vi "RefMem DMA Main Page.vi"(8 "error in (no error)":errorcluster, 11 "Node Ptr":T1 format="%.0x") -> (0 "error out":errorcluster)   [LabVIEW 2015, in "RefMem DMA Custom Device.lvlib"]
uses:
  RefMem DMA Custom Device.lvlib
  <vilib>/NI Veristand/Custom Device API/Custom Device Item Ref.ctl
  <vilib>/NI Veristand/Custom Device API/Custom Device Execution Mode.ctl
  <vilib>/NI Veristand/Custom Device API/Path Specification.ctl
  <vilib>/NI Veristand/Custom Device API/Path Type.ctl
  <vilib>/NI Veristand/Custom Device API/Custom Device Channel.ctl
  <vilib>/NI Veristand/Custom Device API/Custom Device Channel Type.ctl
  Controls/Data Channel Type.ctl
  Reflective Memory File/Reflective Memory File.lvclass
  Controls/Global.vi
  <vilib>/NI Veristand/Custom Device API/Get Item Property (String).vi
  <vilib>/NI Veristand/Custom Device API/Set Item Property (String).vi
  <vilib>/NI Veristand/Custom Device API/Get Item Property (I32).vi
  <vilib>/NI Veristand/Custom Device API/Set Item Property (I32).vi
  <vilib>/NI Veristand/Custom Device API/Set Item Property (U16).vi
  <vilib>/NI Veristand/Custom Device API/Set Item Property (U32).vi
  <vilib>/NI Veristand/Custom Device API/Custom Device API.lvlib
  <vilib>/NI/NI VeriStand Custom Device Import and Export Tool/ImportExport.lvlib
panel:
  out "Path":string
  in  "CPU Assignment":i32
  in  "Import":bool
  in  "Decimation":i32=1 min=1
  in  "VISA Name":string
  in  "Add Data Channel":bool
  in  "Add Data Folder":bool
  in  "Header":cluster{"Section Name":string}={"Section Name"="Reflective Memory Settings"}
  in  "Description":string
  in  "Name":string
  # "(-2 is Automatic)"
  # "Valid values -2, 0, 1.."
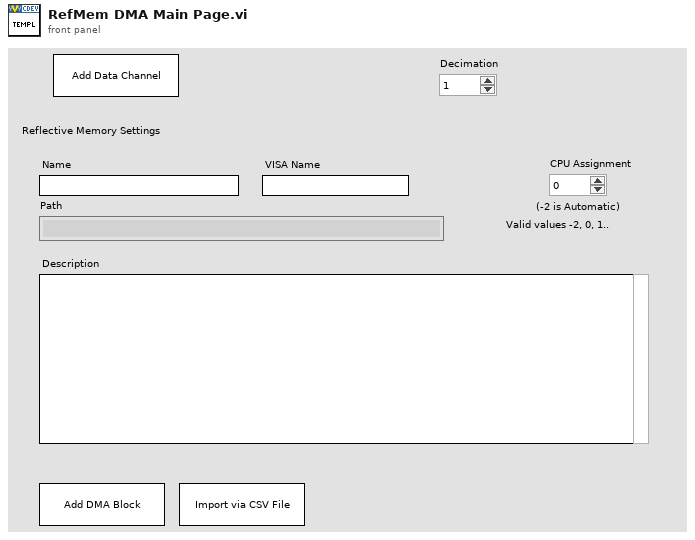
[diagram p1: front panel]
types:
  T1 = typedef "Custom Device API.lvlib/Custom Device Item Ref.ctl" = u64
  T2 = enum8{"Enabled", "Disabled", "Disabled and Grayed Out"}
  T3 = typedef "Custom Device API.lvlib/Custom Device Item Info.ctl" = cluster{"Name":string, "Is Channel":bool, "GUID":string, "Is Waveform":bool}
  T4 = typedef "Custom Device API.lvlib/Path Specification.ctl" = cluster{"Path":path, "Type":T5}
  T5 = typedef "Custom Device API.lvlib/Path Type.ctl" = enum16{"Absolute", "To Base", "To Common Data Dir", "To Application Data Dir"}
  T6 = typedef "Custom Device API.lvlib/Custom Device Execution Mode.ctl" = enum16{"Asynchronous", "Inline HW Interface", "Inline Model Interface", "Inline Timing and Sync", "Asynchronous Timing and Sync"}
  T7 = typedef "RefMem DMA Custom Device.lvlib/Data Channel Type.ctl" = enum16{"Read", "Write"}
  T8 = typedef "Custom Device API.lvlib/Custom Device Channel.ctl" = cluster{"Type":T9, "Units":string, "Default Value":dbl, "Faultable":bool, "Scalable":bool}
  T9 = typedef "Custom Device API.lvlib/Custom Device Channel Type.ctl" = enum16{"Input", "Output"}
  T10 = typedef "Custom Device API.lvlib/Custom Device Commands.ctl" = enum16{"Default", "Item renamed", "Shutdown", "Dynamic button pressed"}
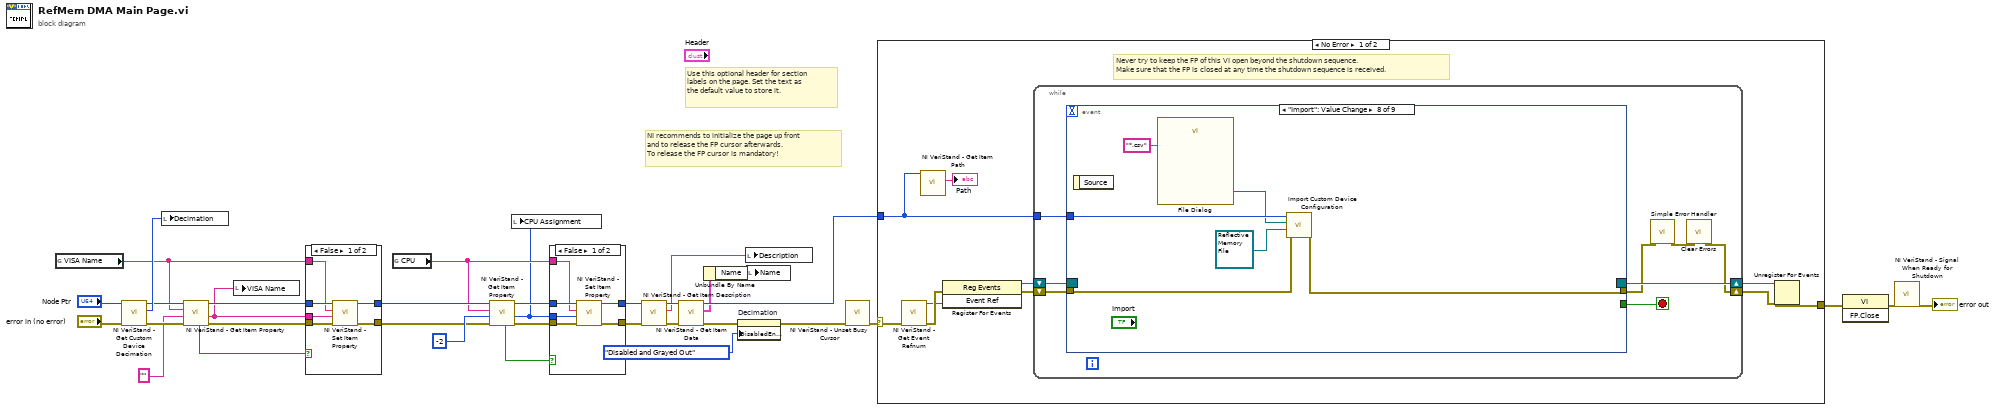
[diagram p0: block diagram]
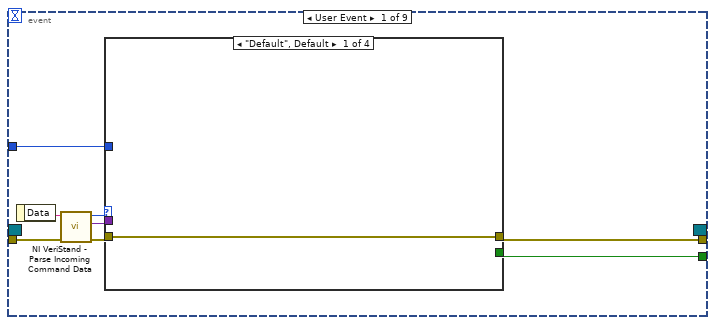
[diagram p4: hidden frame]
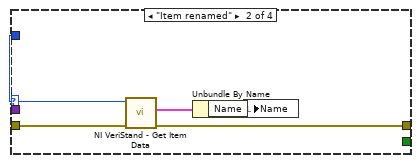
[diagram p5: hidden frame]
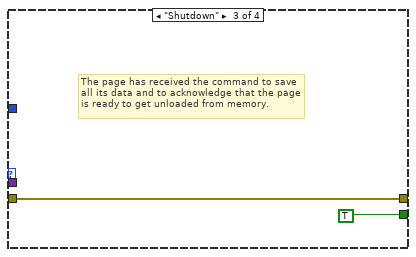
[diagram p6: hidden frame]
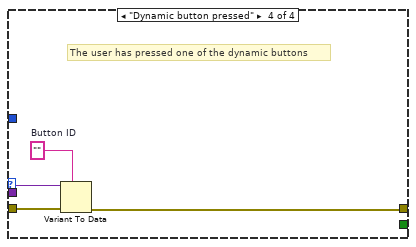
[diagram p7: hidden frame]
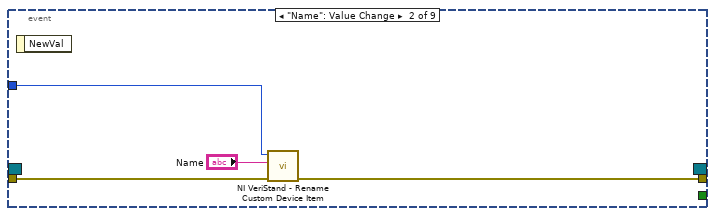
[diagram p8: hidden frame]
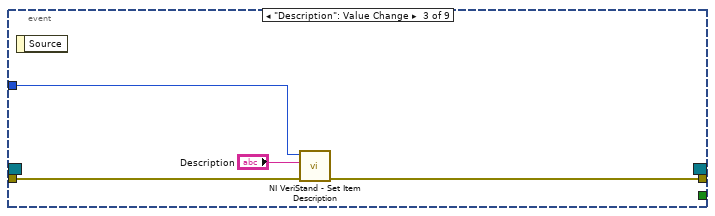
[diagram p9: hidden frame]
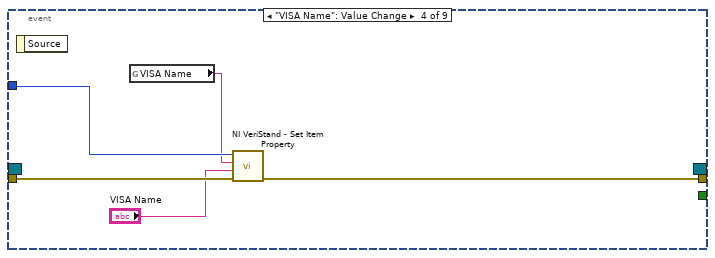
[diagram p10: hidden frame]
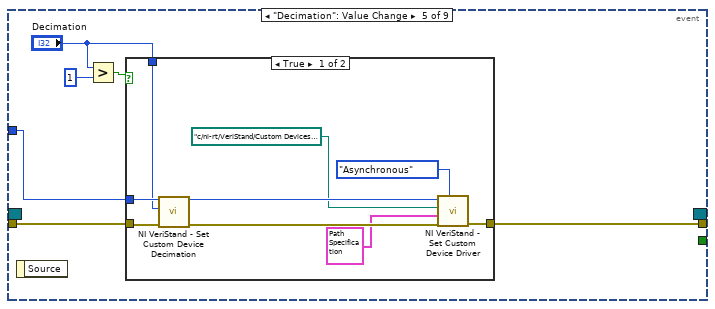
[diagram p11: hidden frame]
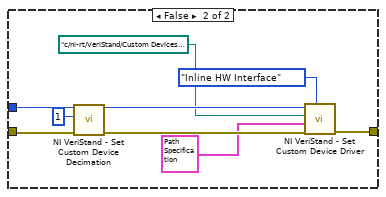
[diagram p12: hidden frame]
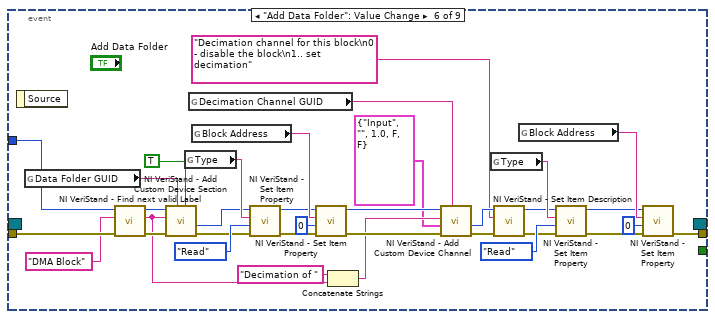
[diagram p13: hidden frame]
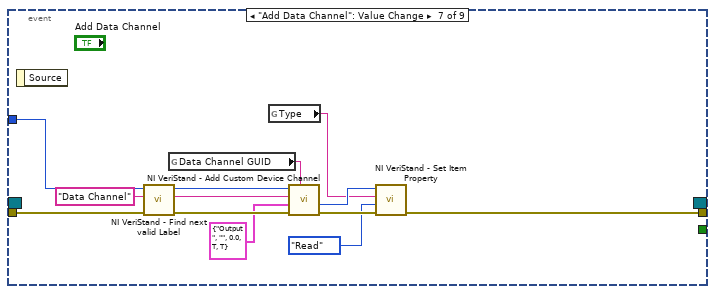
[diagram p14: hidden frame]
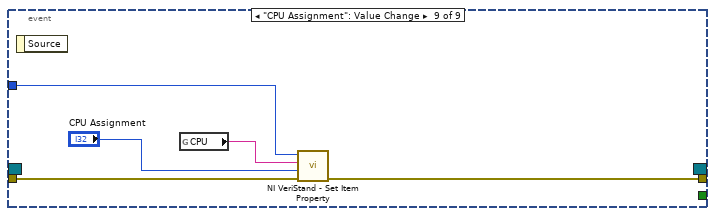
[diagram p15: hidden frame]
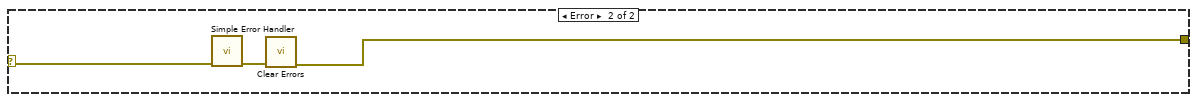
[diagram p16: hidden frame]
diagram:
  # "Use this optional header for section labels on the page. Set the text as the default value to store it."
  # "NI recommends to initialize the page up front\nand to release the FP cursor afterwards.\nTo release the FP cursor is mandatory!"
  n1 = global read "Global.vi" "VISA Name"() -> (w12:string)
  n2 = call <vilib>:"NI VeriStand - Get Custom Device Decimation.vi"("error in (no error)"="error in (no error)", "Device Ref in"="Node Ptr") -> ("error out"=w21:errorcluster, "Decimation"=w22:i32, "Device Ref out"=w20:T1)  [unwired: 7 in]
  n3 = local write "Decimation"(w22) -> ()
  n4 = call-poly <vilib>:"NI VeriStand - Get Item Property.vi"("error in (no error)"=w21, "Default Value"="" ("Section Name"), "Property Name"=w12, "Item Ref in"=w20) -> ("error out"=w10:errorcluster, "Value"=w11:string, "Item Ref out"=w13:T1, "Found?"=w14:bool)  [unwired: 4 in]
  n5 = local write "VISA Name"(w11) -> ()
  n6 = case shown="False" w14 {
    tunnel: w13 -> [w40 w41]
    tunnel: w12 -> [w39 _]
    tunnel: w11 -> [w38 _]
    tunnel: w10 -> [w37 w42]
    tunnel: [w36 w42] -> w9
    tunnel: [w35 w41] -> w8
    frame False {
      n7 = call-poly <vilib>:"NI VeriStand - Set Item Property.vi"("error in (no error)"=w37, "Value"=w38, "Property Name"=w39, "Item Ref in"=w40) -> ("error out"=w36:errorcluster, "Item Ref out"=w35:T1)  [unwired: 5 in, 1 out]
    }
    frame True {
    }
  }
  n8 = global read "Global.vi" "CPU"() -> (w5:string)
  n9 = call-poly <vilib>:"NI VeriStand - Get Item Property.vi"("error in (no error)"=w9, "Default Value"=-2 ("CPU Assignment"), "Property Name"=w5, "Item Ref in"=w8) -> ("error out"=w6:errorcluster, "Value"=w4:i32, "Item Ref out"=w7:T1, "Found?"=w1:bool)  [unwired: 4 in]
  n10 = local write "CPU Assignment"(w4) -> ()
  n11 = case shown="False" w1 {
    tunnel: w7 -> [w48 w49]
    tunnel: w5 -> [w47 _]
    tunnel: w6 -> [w46 w50]
    tunnel: [w45 w50] -> w2
    tunnel: [w44 w49] -> w3
    tunnel: w4 -> [w43 _]
    frame False {
      n12 = call-poly <vilib>:"NI VeriStand - Set Item Property.vi"("error in (no error)"=w46, "Value"=w43, "Property Name"=w47, "Item Ref in"=w48) -> ("error out"=w45:errorcluster, "Item Ref out"=w44:T1)  [unwired: 5 in, 1 out]
    }
    frame True {
    }
  }
  n13 = call <vilib>:"NI VeriStand - Get Item Description.vi"("error in (no error)"=w2, "Item Ref in"=w3) -> ("error out"=w27:errorcluster, "Description"=w28:string, "Item Ref out"=w29:T1)  [unwired: 7 out]
  n14 = call <vilib>:"NI VeriStand - Get Item Data.vi"("error in (no error)"=w27, "Item Ref in"=w29) -> ("error out"=w17:errorcluster, "Item Info"=w26:T3, "Item Ref out"=w30:T1)  [unwired: 7 out]
  n15 = Unbundle By Name(w26) -> ("Name"=w25:string)
  n16 = property on="Decimation" class="DigNum (strict)"(error in=w17, "DisabledEnum"=T2."Disabled and Grayed Out" ("Disabled")) -> (error out=w16:errorcluster)  [unwired: 1 in, 1 out]
  n17 = local write "Description"(w28) -> ()
  n18 = local write "Name"(w25) -> ()
  n19 = call <vilib>:"NI VeriStand - Unset Busy Cursor.vi"("error in (no error)"=w16) -> ("error out"=w31:errorcluster)  [unwired: 10 out]
  n20 = case shown="No Error" w31 {
    selector: w31 -> [w53 w186]
    tunnel: [w57 w184] -> w34
    tunnel: w30 -> [w52 _]
    frame No Error {
      # "Never try to keep the FP of this VI open beyond the shutdown sequence.\nMake sure that the FP is closed at any time the shutdown sequence is received."
      n21 = call <vilib>:"NI VeriStand - Get Event Refnum.vi"("error in (no error)"=w53) -> ("error out"=w60:errorcluster, "Event Ref"=w56:refnum<user-event>)  [unwired: 9 out]
      n22 = call <vilib>:"NI VeriStand - Get Item Path.vi"("Item Ref in"=w52) -> ("Path"=→"Path":string)  [unwired: 7 in, 3 out]
      n23 = register-events(error in=w60, w56) -> (reference out=w54:refnum<event-registration>, error out=w55:errorcluster)  [unwired: 1 in]
      n24 = while {
        tunnel: w52 -> [w64]
        shift-right: [w61] -> w58
        shift-left: w55 -> [w67]
        shift-right: [w68] -> w59
        shift-left: w54 -> [w66]
        stop <- w65 stop-if-true
        n25 = event shown="[7] \"Import\": Value Change" {
          selector: w66 -> [_ _ _ _ _ _ _ _ _]
          dyn-events: [_ _ _ _ _ _ _ _ _] -> w68
          timeout: _ -> [_ _ _ _ _ _ _ _ _]
          tunnel: w67 -> [w76 w92 w95 w101 w105 w158 w171 w177 w183]
          tunnel: [w72 _ _ _ _ _ _ _ _] -> w65
          tunnel: [w71 w91 w94 w99 w104 w126 w163 w176 w182] -> w63
          tunnel: w64 -> [w70 w90 w96 w100 w103 w157 w170 w178 w180]
          event User Event {
            n26 = event-data() -> ("Data"=w75:string)  [unwired: 1 out]
            n27 = call <vilib>:"NI VeriStand - Parse Incoming Command Data.vi"("error in (no error)"=w76, "Incoming data"=w75) -> ("error out"=w74:errorcluster, "Outgoing data"=w69:variant, "Action"=w73:T10)  [unwired: 7 out]
            n28 = case shown="\"Default\", Default" w73 {
              tunnel: w74 -> [w77 w82 w83 w88]
              tunnel: [_ _ TRUE _] -> w72
              tunnel: [w77 w79 w83 w85] -> w71
              tunnel: w70 -> [_ w81 _ _]
              tunnel: w69 -> [_ _ _ w87]
              frame "Default", Default {
              }
              frame "Item renamed" {
                n29 = call <vilib>:"NI VeriStand - Get Item Data.vi"("error in (no error)"=w82, "Item Ref in"=w81) -> ("error out"=w79:errorcluster, "Item Info"=w80:T3)  [unwired: 8 out]
                n30 = Unbundle By Name(w80) -> ("Name"=w78:string)
                n31 = local write "Name"(w78) -> ()
              }
              frame "Shutdown" {
                # "The page has received the command to save all its data and to acknowledge that the page is ready to get unloaded from memory."
              }
              frame "Dynamic button pressed" {
                w86 = ""  # Button ID
                # "The user has pressed one of the dynamic buttons"
                n32 = Variant To Data(error in=w88, type=w86, Variant=w87) -> (error out=w85:errorcluster)  [unwired: 1 out]
              }
            }
          }
          event "Name": Value Change {
            n33 = event-data() -> ()  [unwired: 2 out]
            n34 = call <vilib>:"NI VeriStand - Rename Custom Device Item.vi"("error in (no error)"=w92, "New Name"="Name", "Item Ref in"=w90) -> ("error out"=w91:errorcluster)  [unwired: 1 in, 7 out]
          }
          event "Description": Value Change {
            n35 = event-data() -> ()  [unwired: 2 out]
            n36 = call <vilib>:"NI VeriStand - Set Item Description.vi"("error in (no error)"=w95, "Description"="Description", "Item Ref in"=w96) -> ("error out"=w94:errorcluster)  [unwired: 8 out]
          }
          event "VISA Name": Value Change {
            n37 = event-data() -> ()  [unwired: 2 out]
            n38 = global read "Global.vi" "VISA Name"() -> (w97:string)
            n39 = call-poly <vilib>:"NI VeriStand - Set Item Property.vi"("error in (no error)"=w101, "Value"="VISA Name", "Property Name"=w97, "Item Ref in"=w100) -> ("error out"=w99:errorcluster)  [unwired: 5 in, 2 out]
          }
          event "Decimation": Value Change {
            n40 = event-data() -> ()  [unwired: 2 out]
            n41 = Greater?(x="Decimation", y=u32 1) -> (0:w106:bool)
            n42 = case shown="True" w106 {
              tunnel: w105 -> [w114 w123]
              tunnel: [w116 w125] -> w104
              tunnel: w103 -> [w113 w122]
              tunnel: "Decimation" -> [w112 _]
              frame True {
                n43 = call <vilib>:"NI VeriStand - Set Custom Device Decimation.vi"("error in (no error)"=w114, "Decimation"=w112, "Device Ref in"=w113) -> ("error out"=w111:errorcluster, "Device Ref out"=w110:T1)  [unwired: 7 in]
                n44 = call <vilib>:"NI VeriStand - Set Custom Device Driver.vi"("Execution mode"=Custom_Device_Execution_Mode."Asynchronous", "error in (no error)"=w111, "Driver VI Path (Host)"=T4 {"Path"=path "Custom Devices/RefMem PtByPt/RefMem PtByPt Engine.llb/RefMem PtByPt RT Driver VI (Async).vi", "Type"=enum."To Common Data Dir"}, "Driver VI Path (RT)"=path "c:/ni-rt/VeriStand/Custom Devices/RefMem PtByPt/RefMem PtByPt Engine.llb/RefMem PtByPt RT Driver VI (Async).vi", "Device Ref in"=w110) -> ("error out"=w116:errorcluster)  [unwired: 5 in, 1 out]
              }
              frame False {
                n45 = call <vilib>:"NI VeriStand - Set Custom Device Decimation.vi"("error in (no error)"=w123, "Decimation"=1, "Device Ref in"=w122) -> ("error out"=w121:errorcluster, "Device Ref out"=w120:T1)  [unwired: 7 in]
                n46 = call <vilib>:"NI VeriStand - Set Custom Device Driver.vi"("Execution mode"=Custom_Device_Execution_Mode."Inline HW Interface", "error in (no error)"=w121, "Driver VI Path (Host)"=T4 {"Path"=path "Custom Devices/RefMem PtByPt/RefMem PtByPt Engine.llb/RefMem PtByPt RT Driver VI (Inline).vi", "Type"=enum."To Common Data Dir"}, "Driver VI Path (RT)"=path "c:/ni-rt/VeriStand/Custom Devices/RefMem PtByPt/RefMem PtByPt Engine.llb/RefMem PtByPt RT Driver VI (Inline).vi", "Device Ref in"=w120) -> ("error out"=w125:errorcluster)  [unwired: 5 in, 1 out]
              }
            }
          }
          event "Add Data Folder": Value Change {
            n47 = event-data() -> ()  [unwired: 2 out]
            n48 = global read "Global.vi" "Data Folder GUID"() -> (w159:string)
            n49 = call <vilib>:"NI VeriStand - Find next valid Label.vi"("error in (no error)"=w158, "Label"="DMA Block" ("Section Name"), "Item Ref in"=w157) -> ("error out"=w154:errorcluster, "Label out"=w142:string, "Item Ref out"=w156:T1)  [unwired: 4 in, 2 out]
            n50 = call <vilib>:"NI VeriStand - Add Custom Device Section.vi"("Highlight? (F)"=TRUE, "GUID (Default Section)"=w159, "error in (no error)"=w154, "Section Name"=w142, "Parent Ref in"=w156) -> ("error out"=w150:errorcluster, "Section Ptr"=w145:T1)  [unwired: 3 in, 2 out]
            n51 = global read "Global.vi" "Type"() -> (w152:string)
            n52 = global read "Global.vi" "Decimation Channel GUID"() -> (w140:string)
            n53 = global read "Global.vi" "Block Address"() -> (w153:string)
            n54 = call-poly <vilib>:"NI VeriStand - Set Item Property.vi"("error in (no error)"=w150, "Value"=Data_Channel_Type."Read" ("Type"), "Property Name"=w152, "Item Ref in"=w145) -> ("error out"=w148:errorcluster, "Item Ref out"=w147:T1)  [unwired: 5 in, 1 out]
            n55 = call-poly <vilib>:"NI VeriStand - Set Item Property.vi"("error in (no error)"=w148, "Value"=u32 0 ("Default Value"), "Property Name"=w153, "Item Ref in"=w147) -> ("error out"=w146:errorcluster, "Item Ref out"=w144:T1)  [unwired: 5 in, 1 out]
            n56 = Concatenate Strings("Decimation of " ("string"), w142) -> (w141:string)
            n57 = call <vilib>:"NI VeriStand - Add Custom Device Channel.vi"("GUID (Default Channel)"=w140, "error in (no error)"=w146, "Channel"=T8 {"Type"=enum."Input", "Units"="", "Default Value"=1.0, "Faultable"=FALSE, "Scalable"=FALSE}, "Channel Name"=w141, "Parent Ref in"=w144) -> ("error out"=w138:errorcluster, "Channel Ref"=w137:T1)  [unwired: 3 in, 2 out]
            n58 = global read "Global.vi" "Type"() -> (w133:string)
            n59 = call <vilib>:"NI VeriStand - Set Item Description.vi"("error in (no error)"=w138, "Description"="Decimation channel for this block\n0 - disable the block\n1.. set decimation" ("Section Name"), "Item Ref in"=w137) -> ("error out"=w132:errorcluster, "Item Ref out"=w131:T1)  [unwired: 6 in, 1 out]
            n60 = global read "Global.vi" "Block Address"() -> (w129:string)
            n61 = call-poly <vilib>:"NI VeriStand - Set Item Property.vi"("error in (no error)"=w132, "Value"=Data_Channel_Type."Read" ("Type"), "Property Name"=w133, "Item Ref in"=w131) -> ("error out"=w127:errorcluster, "Item Ref out"=w128:T1)  [unwired: 5 in, 1 out]
            n62 = call-poly <vilib>:"NI VeriStand - Set Item Property.vi"("error in (no error)"=w127, "Value"=u32 0 ("Default Value"), "Property Name"=w129, "Item Ref in"=w128) -> ("error out"=w126:errorcluster)  [unwired: 5 in, 2 out]
          }
          event "Add Data Channel": Value Change {
            n63 = event-data() -> ()  [unwired: 2 out]
            n64 = call <vilib>:"NI VeriStand - Find next valid Label.vi"("error in (no error)"=w171, "Label"="Data Channel", "Item Ref in"=w170) -> ("error out"=w167:errorcluster, "Label out"=w169:string, "Item Ref out"=w168:T1)  [unwired: 4 in, 2 out]
            n65 = global read "Global.vi" "Data Channel GUID"() -> (w172:string)
            n66 = global read "Global.vi" "Type"() -> (w161:string)
            n67 = call <vilib>:"NI VeriStand - Add Custom Device Channel.vi"("GUID (Default Channel)"=w172, "error in (no error)"=w167, "Channel"=T8 {"Type"=enum."Output", "Units"="", "Default Value"=0.0, "Faultable"=TRUE, "Scalable"=TRUE}, "Channel Name"=w169, "Parent Ref in"=w168) -> ("error out"=w164:errorcluster, "Channel Ref"=w162:T1)  [unwired: 3 in, 2 out]
            n68 = call-poly <vilib>:"NI VeriStand - Set Item Property.vi"("error in (no error)"=w164, "Value"=Data_Channel_Type."Read" ("Type"), "Property Name"=w161, "Item Ref in"=w162) -> ("error out"=w163:errorcluster)  [unwired: 5 in, 2 out]
          }
          event "Import": Value Change {
            n69 = event-data() -> ()  [unwired: 2 out]
            n70 = call "File Dialog"("pattern (all files)"="*.csv") -> ("selected path"=w173:path)  [unwired: 11 in, 3 out]
            n71 = call <vilib>:"Import Custom Device Configuration.vi"("error in (no error)"=w177, "File Interface (.dat)"=refnum<class "Reflective Memory File.lvclass"> refnum ("RefMem DMA Custom Device.lvlib:Reflective Memory File.lvclass"), "Path"=w173, "NodeID"=w178) -> ("error out"=w176:errorcluster)  [unwired: 5 in, 2 out]
          }
          event "CPU Assignment": Value Change {
            n72 = event-data() -> ()  [unwired: 2 out]
            n73 = global read "Global.vi" "CPU"() -> (w181:string)
            n74 = call-poly <vilib>:"NI VeriStand - Set Item Property.vi"("error in (no error)"=w183, "Value"="CPU Assignment", "Property Name"=w181, "Item Ref in"=w180) -> ("error out"=w182:errorcluster)  [unwired: 5 in, 2 out]
          }
        }
        n75 = call <vilib>:"Simple Error Handler.vi"("error in (no error)"=w63) -> ("error out"=w62:errorcluster)  [unwired: 1 in, 7 out]
        n76 = call <vilib>:"Clear Errors.vi"("error in (no error)"=w62) -> ("error out"=w61:errorcluster)  [unwired: 1 in, 5 out]
      }
      n77 = Unregister For Events(event registration refnum=w59, error in=w58) -> (error out=w57:errorcluster)
    }
    frame Error {
      n78 = call <vilib>:"Simple Error Handler.vi"("error in (no error)"=w186) -> ("error out"=w185:errorcluster)  [unwired: 1 in, 7 out]
      n79 = call <vilib>:"Clear Errors.vi"("error in (no error)"=w185) -> ("error out"=w184:errorcluster)  [unwired: 1 in, 5 out]
    }
  }
  n80 = invoke class="VI" method="FP.Close"(error in=w34) -> (error out=w33:errorcluster)  [unwired: 2 in, 2 out]
  n81 = call <vilib>:"NI VeriStand - Signal When Ready for Shutdown.vi"("error in (no error)"=w33) -> ("error out"=→"error out":errorcluster)  [unwired: 10 out]
